vi "Curvify.vi"(10 "Linearity":dbl, 11 "Numeric in":dbl) -> (3 "Numeric out":dbl)   [LabVIEW 2013]
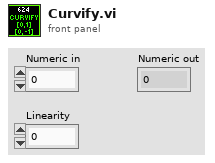
[diagram p1: front panel]
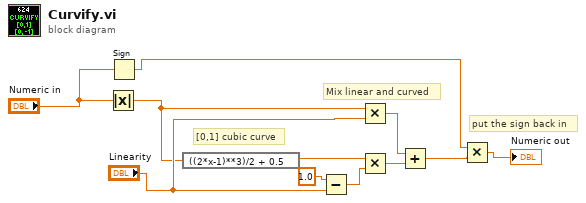
[diagram p0: block diagram]
diagram:
  # "put the sign back in"
  # "Mix linear and curved"
  # "[0,1] cubic curve"
  n1 = Absolute Value(x="Numeric in") -> (abs(x)=w4:dbl)
  n2 = Sign(1:"Numeric in") -> (0:w1:dbl)
  n3 = expression code="((2*x-1)**3)/2 + 0.5"(w4) -> (w6:dbl)
  n4 = Subtract(x=1.0, y="Linearity") -> (x-y=w9:dbl)
  n5 = Multiply(x=w4, y="Linearity") -> (x*y=w11:dbl)
  n6 = Multiply(x=w6, y=w9) -> (x*y=w10:dbl)
  n7 = Add(x=w11, y=w10) -> (x+y=w2:dbl)
  n8 = Multiply(x=w1, y=w2) -> (x*y=→"Numeric out":dbl)
